vi "Gain.vi"(5 "Sample Rate":dbl format="%.2f", 6 "Number of Impulses":i32, 7 "Graph Cluster":T4={"Plot Traces"=[{"Color Box"=4652800, "Boolean"=TRUE, "List 2"=5, "Boolean 2"=FALSE, "Boolean 3"=TRUE, "Offset"=0.0, "Gain"=1.0}, {"Color Box"=16733696, "Boolean"=TRUE, "List 2"=13, "Boolean 2"=TRUE, "Boolean 3"=TRUE, "Offset"=0.0, "Gain"=1.0}, {"Color Box"=393436, "Boolean"=TRUE, "List 2"=21, "Boolean 2"=TRUE, "Boolean 3"=TRUE, "Offset"=0.0, "Gain"=1.0}], "Gain Calculations"={"Threshold Trace"=0, "Min Thresh/%"=0.0, "Max Thresh/%"=0.0, "Gain calculated by dividing"=0, "Gain Range"=enum."Peak %", "Pre-peak-ms"=0.0, "by"=0}, "Impulse Plane"=enum."LARP", "Impulse Direction"=TRUE} {"Gain Calculations"."by" items=["Hx Position-in-Head", "Hy Position-in-Head", "Hz Position-in-Head", "Hx Velocity-in-Head", "Hy Velocity-in-Head", "Hz Velocity-in-Head", "Hl Velocity-in-Head", "Hr Velocity-in-Head", "Lx Position-in-Head", "Ly Position-in-Head", "Lz Position-in-Head", "Lx Velocity-in-Head", "Ly Velocity-in-Head", "Lz Velocity-in-Head", "Ll Velocity-in-Head", "Lr Velocity-in-Head", "Rx Position-in-Head", "Ry Position-in-Head", "Rz Position-in-Head", "Rx Velocity-in-Head", "Ry Velocity-in-Head", "Rz Velocity-in-Head", "Rl Velocity-in-Head", "Rr Velocity-in-Head", "Button", "Ascension X", "Ascension X Vel", "Ascension Y", "Ascension Y Vel", "Ascension Z", "Ascension Z Vel", " "]; "Gain Calculations"."Pre-peak-ms" format="%.2f"; "Gain Calculations"."Gain calculated by dividing" items=["Hx Position-in-Head", "Hy Position-in-Head", "Hz Position-in-Head", "Hx Velocity-in-Head", "Hy Velocity-in-Head", "Hz Velocity-in-Head", "Hl Velocity-in-Head", "Hr Velocity-in-Head", "Lx Position-in-Head", "Ly Position-in-Head", "Lz Position-in-Head", "Lx Velocity-in-Head", "Ly Velocity-in-Head", "Lz Velocity-in-Head", "Ll Velocity-in-Head", "Lr Velocity-in-Head", "Rx Position-in-Head", "Ry Position-in-Head", "Rz Position-in-Head", "Rx Velocity-in-Head", "Ry Velocity-in-Head", "Rz Velocity-in-Head", "Rl Velocity-in-Head", "Rr Velocity-in-Head", "Button", "Ascension X", "Ascension X Vel", "Ascension Y", "Ascension Y Vel", "Ascension Z", "Ascension Z Vel", " "]; "Gain Calculations"."Max Thresh/%" format="%.2f"; "Gain Calculations"."Min Thresh/%" format="%.2f"; "Gain Calculations"."Threshold Trace" items=["Hx Position-in-Head", "Hy Position-in-Head", "Hz Position-in-Head", "Hx Velocity-in-Head", "Hy Velocity-in-Head", "Hz Velocity-in-Head", "Hl Velocity-in-Head", "Hr Velocity-in-Head", "Lx Position-in-Head", "Ly Position-in-Head", "Lz Position-in-Head", "Lx Velocity-in-Head", "Ly Velocity-in-Head", "Lz Velocity-in-Head", "Ll Velocity-in-Head", "Lr Velocity-in-Head", "Rx Position-in-Head", "Ry Position-in-Head", "Rz Position-in-Head", "Rx Velocity-in-Head", "Ry Velocity-in-Head", "Rz Velocity-in-Head", "Rl Velocity-in-Head", "Rr Velocity-in-Head", "Button", "Ascension X", "Ascension X Vel", "Ascension Y", "Ascension Y Vel", "Ascension Z", "Ascension Z Vel", " "]; "Plot Traces"."Gain" format="%.1f"; "Plot Traces"."Offset" format="%.1f"; "Plot Traces"."List 2" items=["Hx Position-in-Head", "Hy Position-in-Head", "Hz Position-in-Head", "Hx Velocity-in-Head", "Hy Velocity-in-Head", "Hz Velocity-in-Head", "Hl Velocity-in-Head", "Hr Velocity-in-Head", "Lx Position-in-Head", "Ly Position-in-Head", "Lz Position-in-Head", "Lx Velocity-in-Head", "Ly Velocity-in-Head", "Lz Velocity-in-Head", "Ll Velocity-in-Head", "Lr Velocity-in-Head", "Rx Position-in-Head", "Ry Position-in-Head", "Rz Position-in-Head", "Rx Velocity-in-Head", "Ry Velocity-in-Head", "Rz Velocity-in-Head", "Rl Velocity-in-Head", "Rr Velocity-in-Head", "Button", "Ascension X", "Ascension X Vel", "Ascension Y", "Ascension Y Vel", "Ascension Z", "Ascension Z Vel", " "]}, 8 "Gain Methods":T3, 9 "Data (in)":dbl[][](array[numeric]) format="%.2f") -> (0 "STD":dbl format="%.2f", 3 "GAIN":dbl format="%.2f")   [LabVIEW 2014, in "generate report.lvlib"]
uses:
  generate report.lvlib
  Enum_Statistical Methods Within Impulses.ctl
  Enum_Statistical Methods Across Impulses.ctl
  <vilib>/Analysis/baseanly.llb/Mean (DBL).vi
  comm/stats/stats.lvlib
  <vilib>/Analysis/NI_AALBase.lvlib
panel:
  # "Copyright Americo A. Migliaccio (c) 2002 All Rights Reserved by Author"
  # "-"
  # "+"
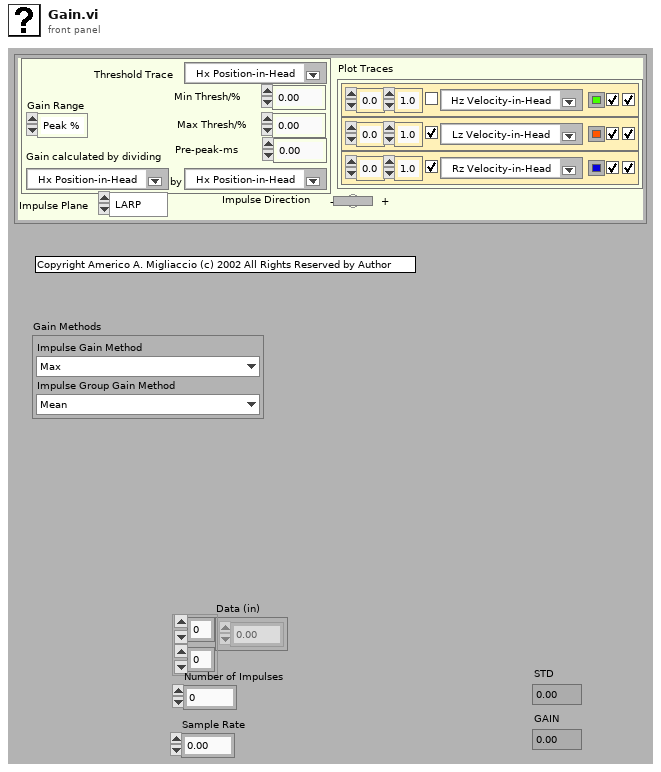
[diagram p1: front panel]
types:
  T1 = typedef "generate report.lvlib/Enum_Statistical Methods Within Impulses.ctl" = enum16{"Max", "Mean", "Median"}
  T2 = typedef "generate report.lvlib/Enum_Statistical Methods Across Impulses.ctl" = enum16{"Mean", "Median"}
  T3 = cluster{"Impulse Gain Method":T1, "Impulse Group Gain Method":T2}
  T4 = cluster{"Plot Traces":cluster{"Color Box":u32, "Boolean":bool, "List 2":u16, "Boolean 2":bool, "Boolean 3":bool, "Offset":dbl, "Gain":dbl}[], "Gain Calculations":cluster{"Threshold Trace":u16, "Min Thresh/%":dbl, "Max Thresh/%":dbl, "Gain calculated by dividing":u16, "Gain Range":enum16{"Peak %", "Best Est", "Thresh"}, "Pre-peak-ms":dbl, "by":u16}, "Impulse Plane":enum16{"Other", "Yaw", "Pitch", "Roll", "LARP", "RALP"}, "Impulse Direction":bool}
  T5 = cluster{"Color Box":u32, "Boolean":bool, "List 2":u16, "Boolean 2":bool, "Boolean 3":bool, "Offset":dbl, "Gain":dbl}[]
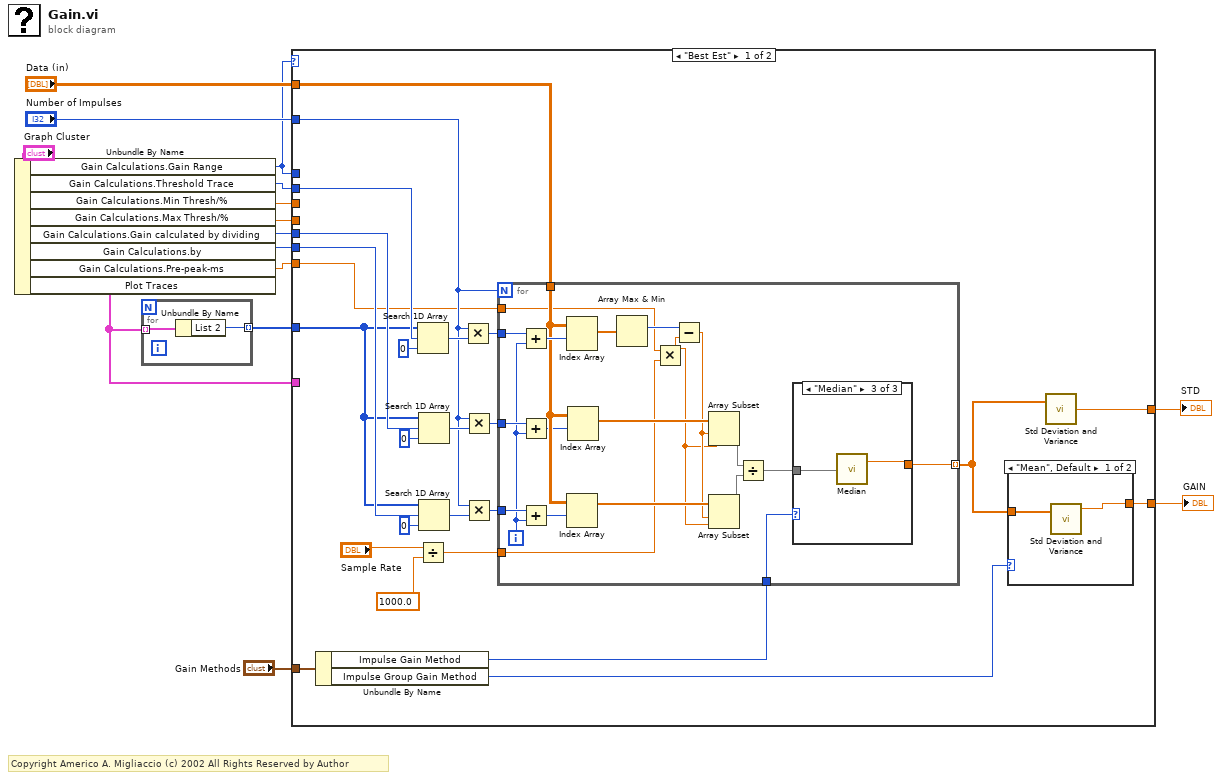
[diagram p0: block diagram]
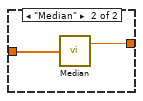
[diagram p2: hidden frame]
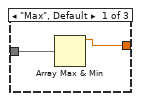
[diagram p3: hidden frame]
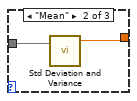
[diagram p4: hidden frame]
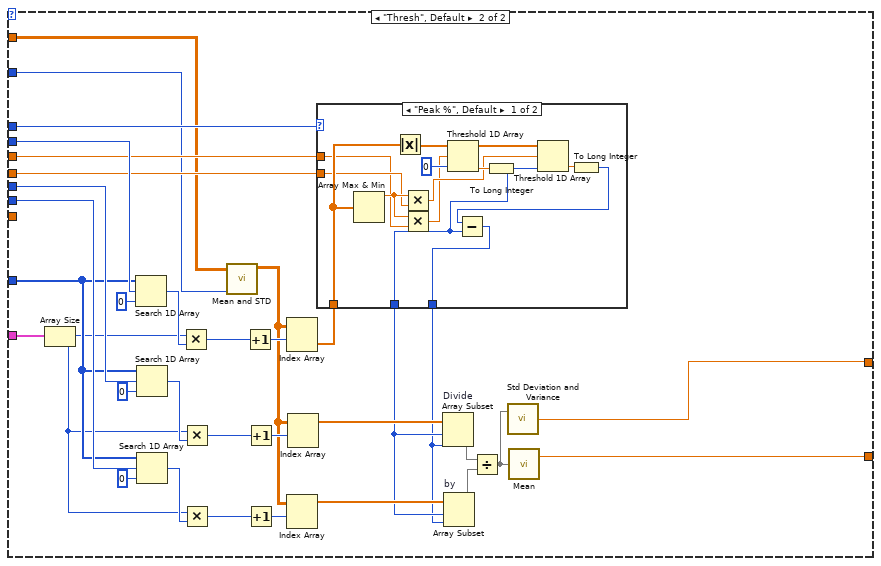
[diagram p5: hidden frame]
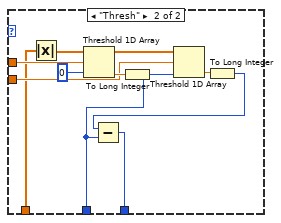
[diagram p6: hidden frame]
diagram:
  # "Copyright Americo A. Migliaccio (c) 2002 All Rights Reserved by Author"
  n1 = Unbundle By Name("Graph Cluster") -> ("Gain Calculations.Gain Range"=w6:enum16{"Peak %", "Best Est", "Thresh"}, "Gain Calculations.Threshold Trace"=w15:u16, "Gain Calculations.Min Thresh/%"=w12:dbl, "Gain Calculations.Max Thresh/%"=w11:dbl, "Gain Calculations.Gain calculated by dividing"=w14:u16, "Gain Calculations.by"=w13:u16, "Gain Calculations.Pre-peak-ms"=w5:dbl, "Plot Traces"=w4:T5)
  n2 = for {
    tunnel: w4 -> [w17] mode=indexing
    tunnel: [w16] -> w8 mode=indexing
    n3 = Unbundle By Name(w17) -> ("List 2"=w16:u16)
  }
  n4 = case shown="\"Best Est\"" w6 {
    tunnel: w15 -> [w32 w107]
    tunnel: w14 -> [w31 w106]
    tunnel: w13 -> [w30 w105]
    tunnel: w12 -> [_ w104]
    tunnel: w11 -> [_ w103]
    tunnel: w6 -> [_ w102]
    tunnel: "Data (in)" -> [w33 w101]
    tunnel: "Number of Impulses" -> [w28 w100]
    tunnel: w8 -> [w29 w93]
    tunnel: w4 -> [_ w78]
    tunnel: [w18 w76] -> w7
    tunnel: w5 -> [w27 _]
    tunnel: [w21 w74] -> w2
    tunnel: "Gain Methods" -> [w23 _]
    frame "Best Est" {
      n5 = Unbundle By Name(w23) -> ("Impulse Gain Method"=w22:T1, "Impulse Group Gain Method"=w19:T2)
      n6 = Search 1D Array(1D array=w29, element=w32, start index (0)=0) -> (index of element=w41:i32)
      n7 = Divide(x="Sample Rate", y=1000.0) -> (x/y=w24:dbl)
      n8 = Search 1D Array(1D array=w29, element=w31, start index (0)=0) -> (index of element=w40:i32)
      n9 = Search 1D Array(1D array=w29, element=w30, start index (0)=0) -> (index of element=w37:i32)
      n10 = Multiply(x=w28, y=w41) -> (x*y=w36:i32)
      n11 = Multiply(x=w28, y=w40) -> (x*y=w35:i32)
      n12 = Multiply(x=w28, y=w37) -> (x*y=w34:i32)
      n13 = for {
        N: w28 -> [_]
        tunnel: w33 -> [w63]
        tunnel: w36 -> [w65]
        tunnel: w35 -> [w67]
        tunnel: w34 -> [w66]
        tunnel: [w48] -> w20 mode=indexing
        tunnel: w27 -> [w52]
        tunnel: w24 -> [w51]
        tunnel: w22 -> [w47]
        i -> [w60]
        n14 = Add(x=w65, y=w60) -> (x+y=w64:i32)
        n15 = Add(x=w67, y=w60) -> (x+y=w62:i32)
        n16 = Add(x=w66, y=w60) -> (x+y=w61:i32)
        n17 = Index Array(array=w63, index (row)=w64) -> (element=w59:dbl[])  [unwired: 1 in]
        n18 = Index Array(array=w63, index (row)=w61) -> (element=w56:dbl[])  [unwired: 1 in]
        n19 = Index Array(array=w63, index (row)=w62) -> (element=w57:dbl[])  [unwired: 1 in]
        n20 = Array Max & Min(array=w59) -> (max index (indices)=w58:i32)  [unwired: 3 out]
        n21 = Multiply(x=w52, y=w51) -> (x*y=w50:dbl)
        n22 = Subtract(x=w58, y=w50) -> (x-y=w55:dbl)
        n23 = Array Subset(array=w57, index=w55, length=w50) -> (w54:dbl[])
        n24 = Array Subset(array=w56, index=w55, length=w50) -> (w53:dbl[])
        n25 = Divide(x=w54, y=w53) -> (x/y=w49:dbl[])
        n26 = case shown="\"Median\"" w47 {
          tunnel: w49 -> [w69 w71 w73]
          tunnel: [w68 w70 w72] -> w48
          frame "Max", Default {
            n27 = Array Max & Min(array=w69) -> (max value=w68:dbl)  [unwired: 3 out]
          }
          frame "Mean" {
            n28 = call <vilib>:"Std Deviation and Variance.vi"("X"=w71) -> ("mean"=w70:dbl)  [unwired: 1 in, 2 out]
          }
          frame "Median" {
            n29 = call <vilib>:"Median.vi"("X"=w73) -> ("median"=w72:dbl)  [unwired: 1 out]
          }
        }
      }
      n30 = case shown="\"Mean\", Default" w19 {
        tunnel: w20 -> [w44 w46]
        tunnel: [w43 w45] -> w18
        frame "Mean", Default {
          n31 = call <vilib>:"Std Deviation and Variance.vi"("X"=w44) -> ("mean"=w43:dbl)  [unwired: 1 in, 2 out]
        }
        frame "Median" {
          n32 = call <vilib>:"Median.vi"("X"=w46) -> ("median"=w45:dbl)  [unwired: 1 out]
        }
      }
      n33 = call <vilib>:"Std Deviation and Variance.vi"("X"=w20) -> ("standard deviation"=w21:dbl)  [unwired: 1 in, 2 out]
    }
    frame "Thresh", Default {
      n34 = Array Size(array=w78) -> (size(s)=w77:i32)
      n35 = Search 1D Array(1D array=w93, element=w107, start index (0)=0) -> (index of element=w97:i32)
      n36 = Search 1D Array(1D array=w93, element=w106, start index (0)=0) -> (index of element=w96:i32)
      n37 = Search 1D Array(1D array=w93, element=w105, start index (0)=0) -> (index of element=w90:i32)
      n38 = Multiply(x=w77, y=w97) -> (x*y=w99:i32)
      n39 = Multiply(x=w77, y=w96) -> (x*y=w94:i32)
      n40 = Multiply(x=w77, y=w90) -> (x*y=w92:i32)
      n41 = call "Mean and STD.vi"("Data (in)"=w101, "Number of Impulses"=w100) -> ("Mean and STD"=w79:dbl[][])  [unwired: 11 in, 2 out]
      n42 = Increment(x=w99) -> (x+1=w89:i32)
      n43 = Increment(x=w94) -> (x+1=w88:i32)
      n44 = Increment(x=w92) -> (x+1=w87:i32)
      n45 = Index Array(array=w79, index (row)=w89) -> (element=w86:dbl[])  [unwired: 1 in]
      n46 = Index Array(array=w79, index (row)=w87) -> (element=w84:dbl[])  [unwired: 1 in]
      n47 = Index Array(array=w79, index (row)=w88) -> (element=w85:dbl[])  [unwired: 1 in]
      n48 = case shown="\"Peak %\", Default" w102 {
        tunnel: w104 -> [w108 w125]
        tunnel: w103 -> [w109 w124]
        tunnel: w86 -> [w113 w123]
        tunnel: [w115 w122] -> w83
        tunnel: [w114 w121] -> w82
        frame "Peak %", Default {
          n49 = Array Max & Min(array=w113) -> (max value=w112:dbl)  [unwired: 3 out]
          n50 = Absolute Value(x=w113) -> (abs(x)=w120:dbl[])
          n51 = Multiply(x=w112, y=w109) -> (x*y=w111:dbl)
          n52 = Multiply(x=w112, y=w108) -> (x*y=w110:dbl)
          n53 = Threshold 1D Array(1:0 ("start index (0)"), 2:w110, 3:w120) -> (0:w116:dbl)
          n54 = To Long Integer(number=w116) -> (32bit integer=w115:i32)
          n55 = Threshold 1D Array(1:w115, 2:w111, 3:w120) -> (0:w117:dbl)
          n56 = To Long Integer(number=w117) -> (32bit integer=w118:i32)
          n57 = Subtract(x=w118, y=w115) -> (x-y=w114:i32)
        }
        frame "Thresh" {
          n58 = Absolute Value(x=w123) -> (abs(x)=w130:dbl[])
          n59 = Threshold 1D Array(1:0 ("start index (0)"), 2:w125, 3:w130) -> (0:w126:dbl)
          n60 = To Long Integer(number=w126) -> (32bit integer=w122:i32)
          n61 = Threshold 1D Array(1:w122, 2:w124, 3:w130) -> (0:w127:dbl)
          n62 = To Long Integer(number=w127) -> (32bit integer=w128:i32)
          n63 = Subtract(x=w128, y=w122) -> (x-y=w121:i32)
        }
      }
      n64 = Array Subset "Divide"(array=w85, index=w83, length=w82) -> (w81:dbl[])
      n65 = Array Subset "by"(array=w84, index=w83, length=w82) -> (w80:dbl[])
      n66 = Divide(x=w81, y=w80) -> (x/y=w75:dbl[])
      n67 = call <vilib>:"Std Deviation and Variance.vi"("X"=w75) -> ("standard deviation"=w74:dbl)  [unwired: 1 in, 2 out]
      n68 = call-poly <vilib>:"Mean.vi"("X"=w75) -> ("mean"=w76:dbl)  [unwired: 1 out]
    }
  }
  "GAIN" <- w7
  "STD" <- w2
